vi "New Chart Actor.vi"(8 "error in (no error)":errorcluster, 11 "Random Data Queue":refnum<queue>) -> (0 "error out":errorcluster, 3 "Chart Actor out":refnum<class "Chart Actor.lvclass">)   [LabVIEW 2021, in "Chart Actor.lvlib" / "Chart Actor.lvclass"]
uses:
  Chart Actor.lvclass
  Chart Actor.lvclass/Chart Actor.ctl
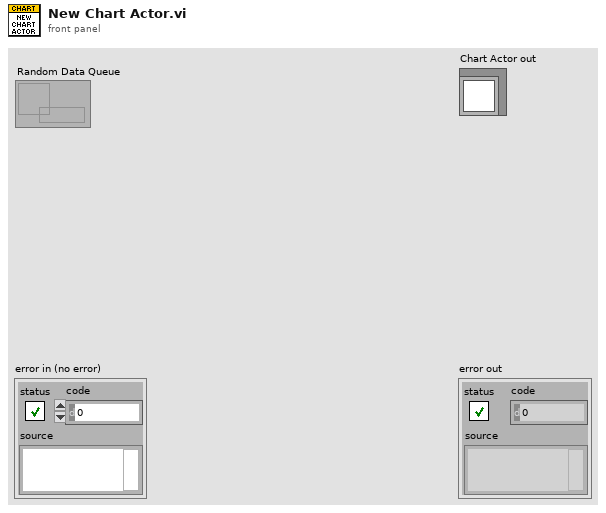
[diagram p1: front panel]
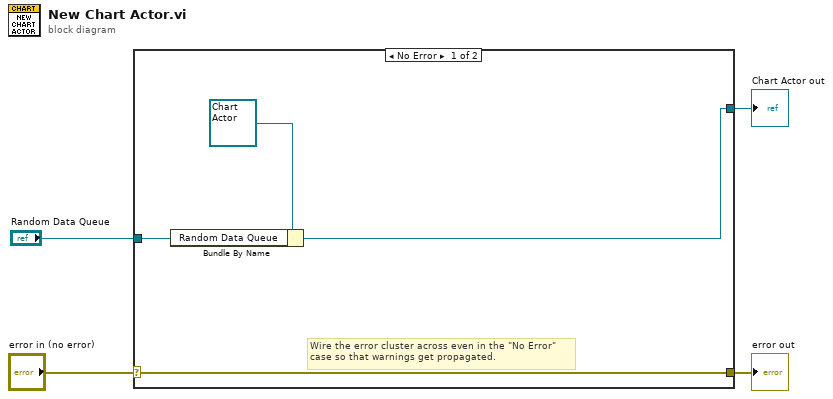
[diagram p0: block diagram]
diagram:
  n1 = case shown="No Error" "error in (no error)" {
    selector: "error in (no error)" -> [w8 w9]
    tunnel: [w8 w9] -> w3
    tunnel: [w6 _] -> w2
    tunnel: "Random Data Queue" -> [w7 _]
    frame No Error {
      # "Wire the error cluster across even in the \"No Error\"\ncase so that warnings get propagated."
      n2 = Bundle By Name(cluster=refnum<class "Chart Actor.lvclass"> refnum ("Chart Actor in"), "Random Data Queue"=w7) -> (w6:refnum<class "Chart Actor.lvclass">)
    }
    frame Error {
    }
  }
  "error out" <- w3
  "Chart Actor out" <- w2
